vi "Xbox Conversion.vi"(1 "Joystick Values":T2) -> (0 "Xbox Values":T1)   [LabVIEW 2014]
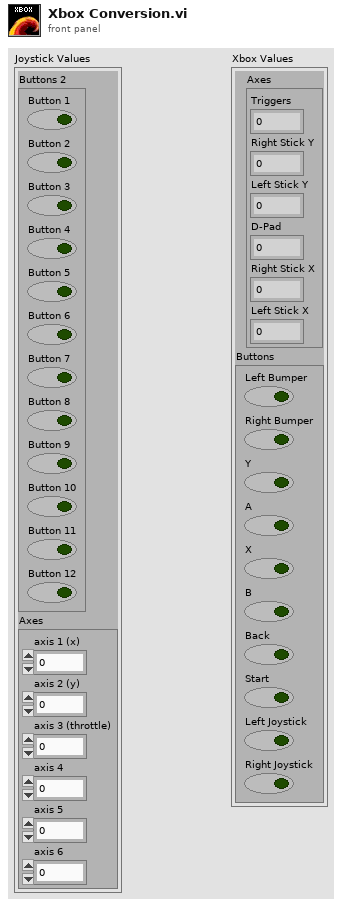
[diagram p1: front panel]
types:
  T1 = cluster{"Axes":cluster{"Triggers":dbl, "Right Stick Y":dbl, "Left Stick Y":dbl, "D-Pad":dbl, "Right Stick X":dbl, "Left Stick X":dbl}, "Buttons":cluster{"Left Bumper":bool, "Right Bumper":bool, "Y":bool, "A":bool, "X":bool, "B":bool, "Back":bool, "Start":bool, "Left Joystick":bool, "Right Joystick":bool}}
  T2 = cluster{"Buttons 2":cluster{"Button 1":bool, "Button 2":bool, "Button 3":bool, "Button 4":bool, "Button 5":bool, "Button 6":bool, "Button 7":bool, "Button 8":bool, "Button 9":bool, "Button 10":bool, "Button 11":bool, "Button 12":bool}, "Axes":cluster{"axis 1 (x)":dbl, "axis 2 (y)":dbl, "axis 3 (throttle)":dbl, "axis 4":dbl, "axis 5":dbl, "axis 6":dbl}}
  T3 = cluster{"Triggers":dbl, "Right Stick Y":dbl, "Left Stick Y":dbl, "D-Pad":dbl, "Right Stick X":dbl, "Left Stick X":dbl}
  T4 = cluster{"Left Bumper":bool, "Right Bumper":bool, "Y":bool, "A":bool, "X":bool, "B":bool, "Back":bool, "Start":bool, "Left Joystick":bool, "Right Joystick":bool}
  T5 = cluster{"Button 1":bool, "Button 2":bool, "Button 3":bool, "Button 4":bool, "Button 5":bool, "Button 6":bool, "Button 7":bool, "Button 8":bool, "Button 9":bool, "Button 10":bool, "Button 11":bool, "Button 12":bool}
  T6 = cluster{"axis 1 (x)":dbl, "axis 2 (y)":dbl, "axis 3 (throttle)":dbl, "axis 4":dbl, "axis 5":dbl, "axis 6":dbl}
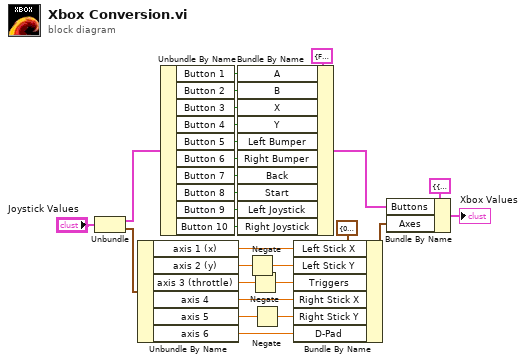
[diagram p0: block diagram]
diagram:
  n1 = Unbundle("Joystick Values") -> ("Buttons 2"=w28:T5, "Axes"=w27:T6)
  n2 = Unbundle By Name(w27) -> ("axis 1 (x)"=w14:dbl, "axis 2 (y)"=w13:dbl, "axis 3 (throttle)"=w12:dbl, "axis 4"=w11:dbl, "axis 5"=w10:dbl, "axis 6"=w9:dbl)
  n3 = Unbundle By Name(w28) -> ("Button 1"=w25:bool, "Button 2"=w24:bool, "Button 3"=w23:bool, "Button 4"=w22:bool, "Button 5"=w21:bool, "Button 6"=w20:bool, "Button 7"=w19:bool, "Button 8"=w18:bool, "Button 9"=w17:bool, "Button 10"=w16:bool)
  n4 = Bundle By Name(cluster=T4 {"Left Bumper"=FALSE, "Right Bumper"=FALSE, "Y"=FALSE, "A"=FALSE, "X"=FALSE, "B"=FALSE, "Back"=FALSE, "Start"=FALSE, "Left Joystick"=FALSE, "Right Joystick"=FALSE}, "A"=w25, "B"=w24, "X"=w23, "Y"=w22, "Left Bumper"=w21, "Right Bumper"=w20, "Back"=w19, "Start"=w18, "Left Joystick"=w17, "Right Joystick"=w16) -> (w6:T4)
  n5 = Negate(x=w13) -> (-x=w3:dbl)
  n6 = Negate(x=w12) -> (-x=w2:dbl)
  n7 = Negate(x=w10) -> (-x=w1:dbl)
  n8 = Bundle By Name(cluster=T3 {"Triggers"=0.0, "Right Stick Y"=0.0, "Left Stick Y"=0.0, "D-Pad"=0.0, "Right Stick X"=0.0, "Left Stick X"=0.0}, "Left Stick X"=w14, "Left Stick Y"=w3, "Triggers"=w2, "Right Stick X"=w11, "Right Stick Y"=w1, "D-Pad"=w9) -> (w5:T3)
  n9 = Bundle By Name(cluster=T1 {"Axes"={"Triggers"=0.0, "Right Stick Y"=0.0, "Left Stick Y"=0.0, "D-Pad"=0.0, "Right Stick X"=0.0, "Left Stick X"=0.0}, "Buttons"={"Left Bumper"=FALSE, "Right Bumper"=FALSE, "Y"=FALSE, "A"=FALSE, "X"=FALSE, "B"=FALSE, "Back"=FALSE, "Start"=FALSE, "Left Joystick"=FALSE, "Right Joystick"=FALSE}}, "Buttons"=w6, "Axes"=w5) -> (→"Xbox Values":T1)
